vi "Main.vi"   [LabVIEW 2016, in "HelloWorld-AF.lvlib"]
doc: "This is the Main.vi of LabVIEW's Hello World based on NI's Actor Framework.\n\nIt launches the GUI-Actor which controls the DAQ, Analysis and Storage."
uses:
  HelloWorld-AF.lvlib
  <vilib>/ActorFramework/Stop Msg/Stop Msg.lvclass/Stop Msg.ctl
  <vilib>/ActorFramework/Message Enqueuer/Message Enqueuer.lvclass/Message Enqueuer.ctl
  Actors/LHW-GUI/LHW-GUI-Actor.lvclass
  C:/Program Files (x86)/National Instruments/LabVIEW 2016/vi.lib/ActorFramework/Actor/Actor.lvclass
  <vilib>/ActorFramework/Message Enqueuer/Enqueue Critical.vi
  <vilib>/ActorFramework/Message Enqueuer/Enqueue.vi
  <vilib>/ActorFramework/Stop Msg/Stop Msg.lvclass
  C:/Program Files (x86)/National Instruments/LabVIEW 2016/vi.lib/ActorFramework/Message/Message.lvclass
  <vilib>/ActorFramework/Message Priority Queue/Priority Enqueue.vi
  <vilib>/ActorFramework/Message Enqueuer/Message Enqueuer.lvclass
  <vilib>/ActorFramework/Actor/Actor.lvclass
panel:
  # "Check menu for possible actions."
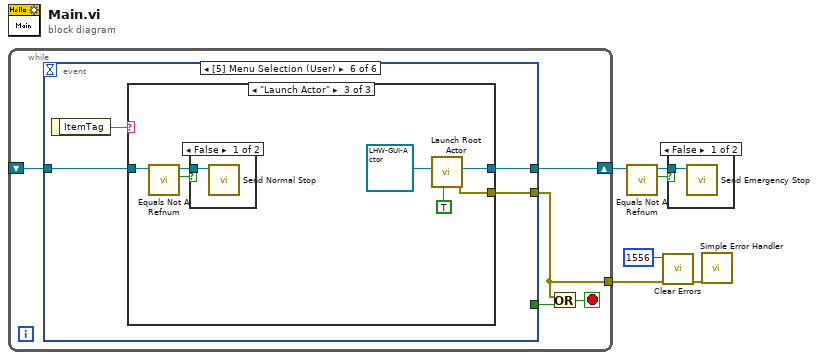
[diagram p0: block diagram]
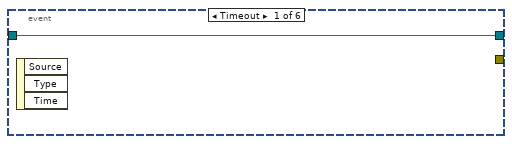
[diagram p3: hidden frame]
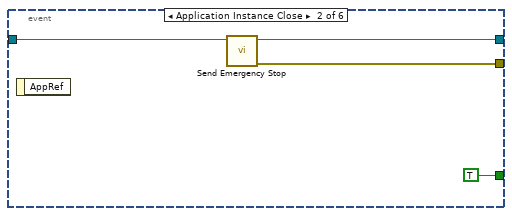
[diagram p4: hidden frame]
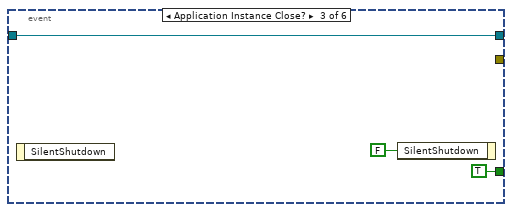
[diagram p5: hidden frame]
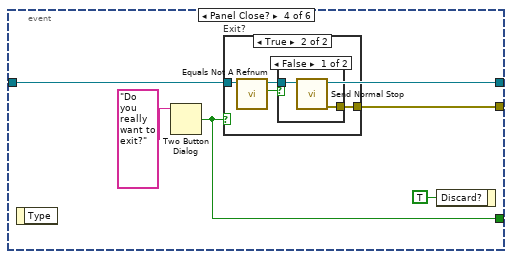
[diagram p6: hidden frame]
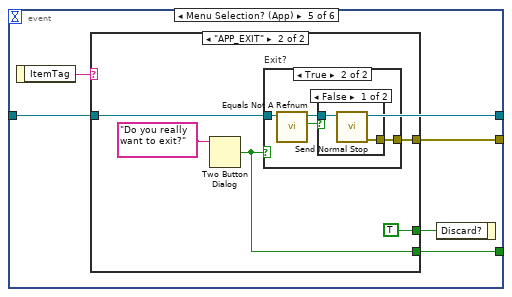
[diagram p9: hidden frame]
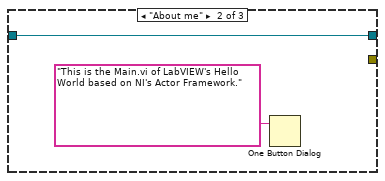
[diagram p14: hidden frame]
diagram:
  n1 = while {
    shift-right: [w6] -> w5
    shift-left: _ -> [w10]
    tunnel: [w7] -> w2
    stop <- w8 stop-if-true
    n2 = event shown="[5] Menu Selection (User)" {
      selector: _ -> [_ _ _ _ _ _]
      dyn-events: _ -> [_ _ _ _ _ _]
      timeout: _ -> [_ _ _ _ _ _]
      tunnel: w10 -> [w11 w12 w15 w19 w30 w44]
      tunnel: [_ w14 _ w18 w29 w43] -> w7
      tunnel: [_ TRUE TRUE w21 w32 _] -> w9
      tunnel: [w11 w12 w15 w19 w30 w45] -> w6
      event Timeout {
        n3 = event-data() -> ()  [unwired: 1 in, 3 out]
      }
      event Application Instance Close {
        n4 = event-data() -> ()  [unwired: 1 in, 1 out]
        n5 = call <vilib>:"Send Emergency Stop.vi"("Message Enqueuer"=w12) -> ("error out"=w14:errorcluster)  [unwired: 10 in]
      }
      event Application Instance Close? {
        n6 = event-data() -> ()  [unwired: 1 in, 1 out]
        n7 = event-data("SilentShutdown"=FALSE) -> ()  [unwired: 1 in, 1 out]
      }
      event Panel Close? {
        n8 = event-data() -> ()  [unwired: 1 in, 1 out]
        n9 = Two Button Dialog(message="Do you really want to exit?") -> (T button?=w21:bool)  [unwired: 2 in]
        n10 = case "Exit?" shown="True" w21 {
          tunnel: w19 -> [_ w24]
          tunnel: [_ w23] -> w18
          frame False {
          }
          frame True {
            n11 = call <vilib>:"Equals Not A Refnum.vi"("Message Enqueuer"=w24) -> ("Not a refnum?"=w25:bool)  [unwired: 10 in]
            n12 = case shown="False" w25 {
              tunnel: w24 -> [w27 _]
              tunnel: [w26 _] -> w23
              frame False {
                n13 = call <vilib>:"Send Normal Stop.vi"("Message Enqueuer"=w27) -> ("error out"=w26:errorcluster)  [unwired: 10 in]
              }
              frame True {
              }
            }
          }
        }
        n14 = event-data("Discard?"=TRUE) -> ()  [unwired: 1 in, 1 out]
      }
      event Menu Selection? (App) {
        n15 = event-data() -> ("ItemTag"=w31:string)  [unwired: 1 in]
        n16 = case shown="\"APP_EXIT\"" w31 {
          tunnel: w30 -> [_ w37]
          tunnel: [_ w36] -> w32
          tunnel: [_ w34] -> w29
          tunnel: [_ TRUE ("Discard?")] -> w28
          frame Default {
          }
          frame "APP_EXIT" {
            n17 = Two Button Dialog(message="Do you really want to exit?") -> (T button?=w36:bool)  [unwired: 2 in]
            n18 = case "Exit?" shown="True" w36 {
              tunnel: w37 -> [_ w39]
              tunnel: [_ w38] -> w34
              frame False {
              }
              frame True {
                n19 = call <vilib>:"Equals Not A Refnum.vi"("Message Enqueuer"=w39) -> ("Not a refnum?"=w40:bool)  [unwired: 10 in]
                n20 = case shown="False" w40 {
                  tunnel: w39 -> [w42 _]
                  tunnel: [w41 _] -> w38
                  frame False {
                    n21 = call <vilib>:"Send Normal Stop.vi"("Message Enqueuer"=w42) -> ("error out"=w41:errorcluster)  [unwired: 10 in]
                  }
                  frame True {
                  }
                }
              }
            }
          }
        }
        n22 = event-data("Discard?"=w28) -> ()  [unwired: 1 in, 1 out]
      }
      event Menu Selection (User) {
        n23 = event-data() -> ("ItemTag"=w46:string)  [unwired: 1 in]
        n24 = case shown="\"Launch Actor\"" w46 {
          tunnel: [w47 w48 w55] -> w45
          tunnel: w44 -> [w47 w48 w54]
          tunnel: [_ _ w52] -> w43
          frame Default {
          }
          frame "About me" {
            n25 = One Button Dialog(message="This is the Main.vi of LabVIEW's Hello World based on NI's Actor Framework.") -> ()  [unwired: 1 in, 1 out]
          }
          frame "Launch Actor" {
            n26 = call <vilib>:"Equals Not A Refnum.vi"("Message Enqueuer"=w54) -> ("Not a refnum?"=w53:bool)  [unwired: 10 in]
            n27 = case shown="False" w53 {
              tunnel: w54 -> [w56 _]
              frame False {
                n28 = call <vilib>:"Send Normal Stop.vi"("Message Enqueuer"=w56) -> ()  [unwired: 10 in, 1 out]
              }
              frame True {
              }
            }
            n29 = call <vilib>:"Launch Root Actor.vi"("Open Actor Core front panel? (F)"=TRUE, "Actor"=refnum<class "LHW-GUI-Actor.lvclass"> refnum ("LHW-GUI.lvlib:LHW-GUI-Actor.lvclass")) -> ("error out"=w52:errorcluster, "Actor's Enqueuer"=w55:refnum<class "Message Enqueuer.lvclass">)  [unwired: 8 in]
          }
        }
      }
    }
    n30 = Or(x=w7, y=w9) -> (x .or. y?=w8:bool)
  }
  n31 = call <vilib>:"Equals Not A Refnum.vi"("Message Enqueuer"=w5) -> ("Not a refnum?"=w4:bool)  [unwired: 10 in]
  n32 = call <vilib>:"Clear Errors.vi"("error in (no error)"=w2, "specific error code to clear (0: all)"=1556) -> ("error out"=w3:errorcluster)  [unwired: 4 in, 1 out]
  n33 = case shown="False" w4 {
    tunnel: w5 -> [w57 _]
    frame False {
      n34 = call <vilib>:"Send Emergency Stop.vi"("Message Enqueuer"=w57) -> ()  [unwired: 10 in, 1 out]
    }
    frame True {
    }
  }
  n35 = call <vilib>:"Simple Error Handler.vi"("error in (no error)"=w3) -> ()  [unwired: 4 in, 5 out]
